vi "myRIO_BRig_Host_endExp_check.vi"() -> (2 "output_IendExp":bool, 3 "output_filePath_expExp":path)   [LabVIEW 2014]
panel:
  out "output_error":errorcluster
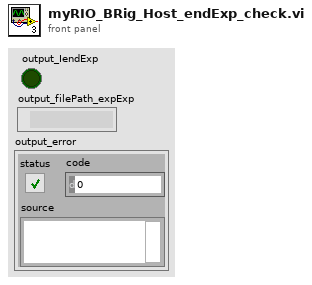
[diagram p1: front panel]
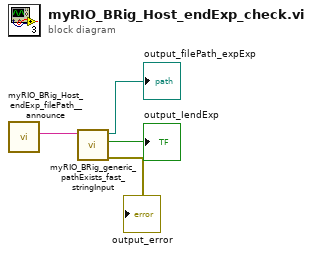
[diagram p0: block diagram]
diagram:
  n1 = call "myRIO_BRig_Host_endExp_filePath__announce.vi"() -> ("concatenated string"=w4:string)  [unwired: 11 in]
  n2 = call "myRIO_BRig_generic_pathExists_fast_stringInput.vi"("input_filePath"=w4) -> ("output_error"=→"output_error":errorcluster, "output_Iexist"=→"output_IendExp":bool, "output_filePath"=→"output_filePath_expExp":path)  [unwired: 8 in]
